vi "GlobalChunkSave_test.vi"(3 "Findex":i32, 5 "length":i32, 6 "Time":timestamp, 7 "index":i32, 8 "Array 2":dbl[](array[numeric]), 9 "Average":dbl, 10 "ChunkDefinition":T1, 11 "mode":enum16{"init", "store", "read"}(ring)) -> (2 "Array":T2(array[cluster]) {"Average" format="%.2f"})   [LabVIEW 2020, in "Sgraph_lib_V1.lvlib"]
uses:
  Builds/Sgraph_lib_V1.lvlib
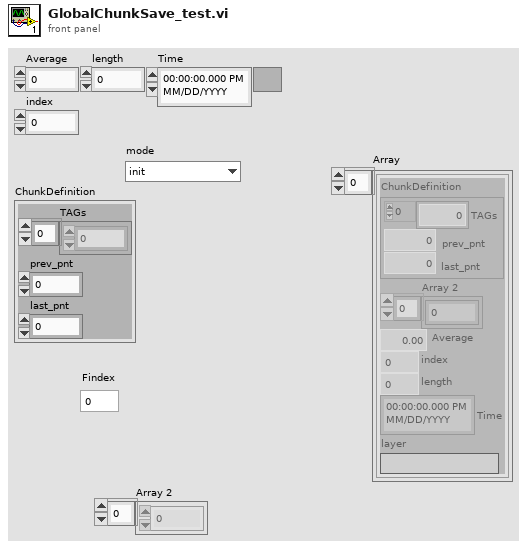
[diagram p1: front panel]
types:
  T1 = cluster{"TAGs":i32[], "prev_pnt":i32, "last_pnt":i32}
  T2 = cluster{"ChunkDefinition":cluster{"TAGs":i32[], "prev_pnt":i32, "last_pnt":i32}, "Array 2":dbl[], "Average":dbl, "index":i32, "length":i32, "Time":timestamp, "layer":string}[]
  T3 = cluster{"ChunkDefinition":cluster{"TAGs":i32[], "prev_pnt":i32, "last_pnt":i32}, "Array 2":dbl[], "Average":dbl, "index":i32, "length":i32, "Time":timestamp, "layer":string}
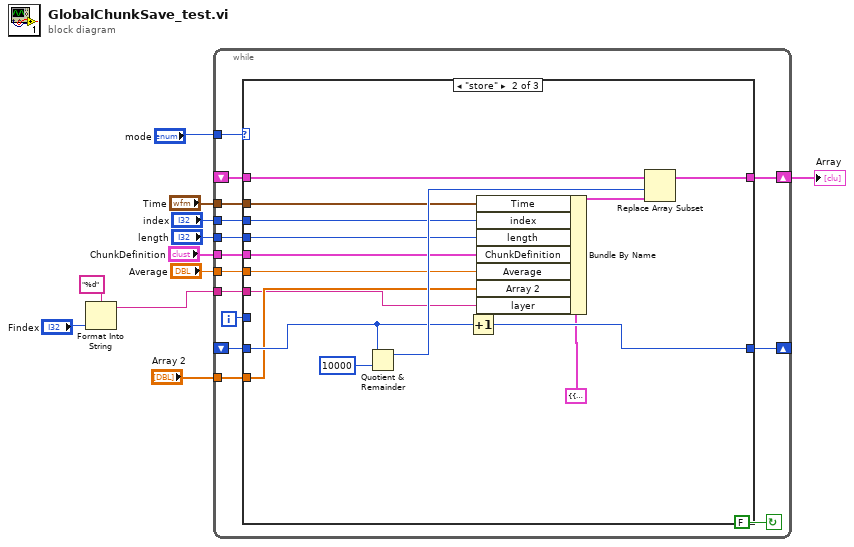
[diagram p0: block diagram]
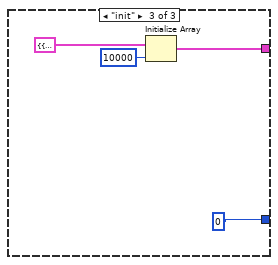
[diagram p3: hidden frame]
diagram:
  n1 = Format Into String(format string="%d", "Findex") -> (resulting string=w2:string)  [unwired: 2 in, 1 out]
  n2 = while {
    tunnel: "mode" -> [w25]
    shift-right: [w24] -> w10
    shift-left: _ -> [w23]
    tunnel: "ChunkDefinition" -> [w21]
    shift-right: [w18] -> _
    shift-left: _ -> [w19]
    tunnel: "Array 2" -> [w17]
    tunnel: "Average" -> [w16]
    tunnel: "index" -> [w15]
    tunnel: "length" -> [w14]
    tunnel: "Time" -> [w13]
    tunnel: w2 -> [w12]
    i -> [w22]
    stop <- FALSE continue-if-true
    n3 = case shown="\"store\"" w25 {
      tunnel: [w27 w39 w46] -> w24
      tunnel: w23 -> [w27 w42 _]
      tunnel: w22 -> [_ _ _]
      tunnel: w21 -> [_ w37 _]
      tunnel: w19 -> [w26 w35 _]
      tunnel: [w26 w36 0 ("y")] -> w18
      tunnel: w17 -> [_ w34 _]
      tunnel: w16 -> [_ w32 _]
      tunnel: w15 -> [_ w31 _]
      tunnel: w14 -> [_ w30 _]
      tunnel: w13 -> [_ w29 _]
      tunnel: w12 -> [_ w28 _]
      frame Default {
      }
      frame "store" {
        n4 = Quotient & Remainder(x=w35, y=10000) -> (x-y*floor(x/y)=w40:i32)  [unwired: 1 out]
        n5 = Increment(x=w35) -> (x+1=w36:i32)
        n6 = Bundle By Name(cluster=T3 {"ChunkDefinition"={"TAGs"=[0, 1, 2, 3, 4, 5, 6, 7, 8, 9, 10, 11, 12, 13, 14, 15, 16, 17, 18, 19, 20, 21, 22, 23, 24, 25, 26, 27, 28, 29, 30, 31, 32, 33, 34, 35, 36, 37, 38, 39, 40, 41, 42, 43, 44, 45, 46, 47, 48, 49, 50, 51, 52, 53, 54, 55, 56, 57, 58, 59, 60, 61, 62, 63, 64, 65, 66, 67, 68, 69, 70, 71, 72, 73, 74, 75, 76, 77, 78, 79, 80, 81, 82, 83, 84, 85, 86, 87, 88, 89, 90, 91, 92, 93, 94, 95, 96, 97, 98, 99], "prev_pnt"=-1, "last_pnt"=0}, "Array 2"=[-0.8968895039512168], "Average"=0.0, "index"=0, "length"=0, "Time"=timestamp(3672569476.1593866 s since 1904-01-01), "layer"=""} ("Cluster"), "Time"=w29, "index"=w31, "length"=w30, "ChunkDefinition"=w37, "Average"=w32, "Array 2"=w34, "layer"=w28) -> (w38:T3)
        n7 = Replace Array Subset(array=w42, new element=w38, index=w40) -> (w39:T2)
      }
      frame "init" {
        n8 = Initialize Array(T3 {"ChunkDefinition"={"TAGs"=[0, 1, 2, 3, 4, 5, 6, 7, 8, 9, 10, 11, 12, 13, 14, 15, 16, 17, 18, 19, 20, 21, 22, 23, 24, 25, 26, 27, 28, 29, 30, 31, 32, 33, 34, 35, 36, 37, 38, 39, 40, 41, 42, 43, 44, 45, 46, 47, 48, 49, 50, 51, 52, 53, 54, 55, 56, 57, 58, 59, 60, 61, 62, 63, 64, 65, 66, 67, 68, 69, 70, 71, 72, 73, 74, 75, 76, 77, 78, 79, 80, 81, 82, 83, 84, 85, 86, 87, 88, 89, 90, 91, 92, 93, 94, 95, 96, 97, 98, 99], "prev_pnt"=-1, "last_pnt"=0}, "Array 2"=[-0.8968895039512168], "Average"=0.0, "index"=0, "length"=0, "Time"=timestamp(3672569476.1593866 s since 1904-01-01), "layer"=""} ("Cluster"), 10000 ("dimension size")) -> (w46:T2)
      }
    }
  }
  "Array" <- w10
